vi "Wait For Motion Stop.vi"(4 "error in (no error)":errorcluster, 5 "delay after motion is complete (0ms)":i32 min=0 max=60000, 6 "Axis (0)":i32 min=0 max=3, 7 "VISA resource name":refnum<visa-resource-name>) -> (0 "error out":errorcluster, 3 "VISA resource name out":refnum<visa-resource-name>)   [LabVIEW 2012, in "Newport ESP301.lvlib"]
doc: "This command stops the program execution until a motion is completed. The\nprogram is continued only after <B>Axis (0)</B> reaches its destination. If <B>Axis (0)</B> is not specified, the controller waits for all motion in progress to end. If <B>delay after motion is complete (0ms)</B> is specified different than 0, the controller waits an additional <B> delay after motion is complete (0ms)</B> milliseconds after the motion is complete and then executes the next commands.\nNote:\nWait commands are primarily intended for use in internal program execution or in combination with the RQ command. If used in command mode, it is important to note that input command processing is suspended until the wait condition has been satisfied."
uses:
  Newport ESP301.lvlib
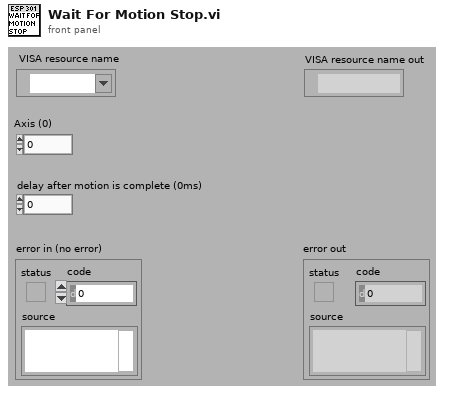
[diagram p1: front panel]
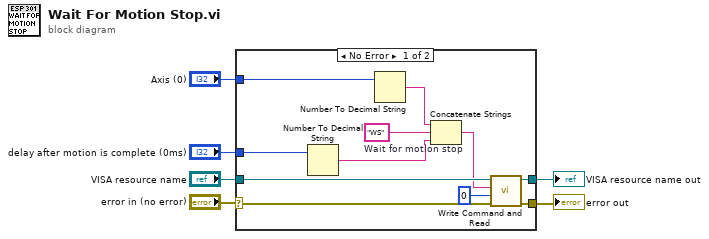
[diagram p0: block diagram]
diagram:
  n1 = case shown="No Error" "error in (no error)" {
    selector: "error in (no error)" -> [w11 w19]
    tunnel: [w9 w19] -> w6
    tunnel: "VISA resource name" -> [w14 w18]
    tunnel: [w10 w18] -> w5
    tunnel: "Axis (0)" -> [w15 _]
    tunnel: "delay after motion is complete (0ms)" -> [w7 _]
    frame No Error {
      w17 = "WS"  # Wait for motion stop
      n2 = Number To Decimal String(number=w7) -> (decimal integer string=w8:string)  [unwired: 1 out]
      n3 = Number To Decimal String(number=w15) -> (decimal integer string=w16:string)  [unwired: 1 out]
      n4 = Concatenate Strings(w16, w17, w8) -> (w13:string)
      n5 = call "Write Command and Read.vi"("error in (no error)"=w11, "Bytes to read (100)"=u32 0, "Command"=w13, "VISA resource name"=w14) -> ("error out"=w9:errorcluster, "VISA resource name out"=w10:refnum<visa-resource-name>)  [unwired: 1 in, 3 out]
    }
    frame Error {
    }
  }
  "error out" <- w6
  "VISA resource name out" <- w5
